vi "TIO Form Packet.vi"(9 "Routing":string="\u0000\u0001", 10 "Type":T1(ring)=enum."RPC Request", 11 "Payload":string="Q\u0017\b€dev.name") -> (3 "String out":string)   [LabVIEW 2010]
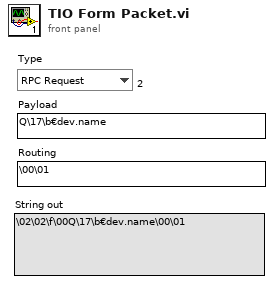
[diagram p1: front panel]
types:
  T1 = enum8{"Invalid", "Log", "RPC Request", "RPC Reply", "RPC Error", "Stream Description", "User"}
  T2 = enum16{"big-endian, network order", "native, host order", "little-endian"}
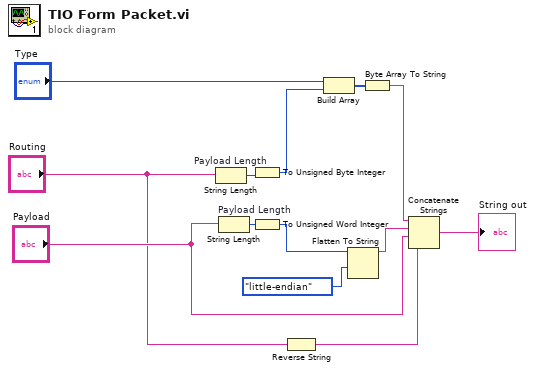
[diagram p0: block diagram]
diagram:
  n1 = String Length "Payload Length"(string="Routing") -> (length=w6:i32)
  n2 = String Length "Payload Length"(string="Payload") -> (length=w8:i32)
  n3 = To Unsigned Byte Integer(number=w6) -> (unsigned 8bit integer=w5:u8)
  n4 = To Unsigned Word Integer(number=w8) -> (unsigned 16bit integer=w10:u16)
  n5 = Reverse String(1:"Routing") -> (0:w1:string)
  n6 = Build Array("Type", w5) -> (w4:u8[])
  n7 = Flatten To String(anything=w10, byte order (0:big-endian, network order)=T2."little-endian") -> (data string=w9:string)  [unwired: 2 in, 2 out]
  n8 = Byte Array To String(unsigned byte array=w4) -> (string=w3:string)
  n9 = Concatenate Strings(w3, w9, "Payload", w1) -> (→"String out":string)
